vi "7SegmentDecoder.vi"() -> ()   [LabVIEW 2022 SP3]
panel:
  out "DH":T1 {"E" scale=0.0..1.0 scale format="%b"; "D" scale=0.0..1.0 scale format="%b"; "C" scale=0.0..1.0 scale format="%b"; "G" scale=0.0..1.0 scale format="%b"; "B" scale=0.0..1.0 scale format="%b"; "A" scale=0.0..1.0 scale format="%b"; "F" scale=0.0..1.0 scale format="%b"}
  out "UH":T1 {"E" scale=0.0..1.0 scale format="%b"; "D" scale=0.0..1.0 scale format="%b"; "C" scale=0.0..1.0 scale format="%b"; "G" scale=0.0..1.0 scale format="%b"; "B" scale=0.0..1.0 scale format="%b"; "A" scale=0.0..1.0 scale format="%b"; "F" scale=0.0..1.0 scale format="%b"}
  out "DM":T1 {"E" scale=0.0..1.0 scale format="%b"; "D" scale=0.0..1.0 scale format="%b"; "C" scale=0.0..1.0 scale format="%b"; "G" scale=0.0..1.0 scale format="%b"; "B" scale=0.0..1.0 scale format="%b"; "A" scale=0.0..1.0 scale format="%b"; "F" scale=0.0..1.0 scale format="%b"}
  out "UM":T1 {"E" scale=0.0..1.0 scale format="%b"; "D" scale=0.0..1.0 scale format="%b"; "C" scale=0.0..1.0 scale format="%b"; "G" scale=0.0..1.0 scale format="%b"; "B" scale=0.0..1.0 scale format="%b"; "A" scale=0.0..1.0 scale format="%b"; "F" scale=0.0..1.0 scale format="%b"}
  out "DS":T1 {"E" scale=0.0..1.0 scale format="%b"; "D" scale=0.0..1.0 scale format="%b"; "C" scale=0.0..1.0 scale format="%b"; "G" scale=0.0..1.0 scale format="%b"; "B" scale=0.0..1.0 scale format="%b"; "A" scale=0.0..1.0 scale format="%b"; "F" scale=0.0..1.0 scale format="%b"}
  in  "stop":bool
  out "US":T1 {"E" scale=0.0..1.0 scale format="%b"; "D" scale=0.0..1.0 scale format="%b"; "C" scale=0.0..1.0 scale format="%b"; "G" scale=0.0..1.0 scale format="%b"; "B" scale=0.0..1.0 scale format="%b"; "A" scale=0.0..1.0 scale format="%b"; "F" scale=0.0..1.0 scale format="%b"}
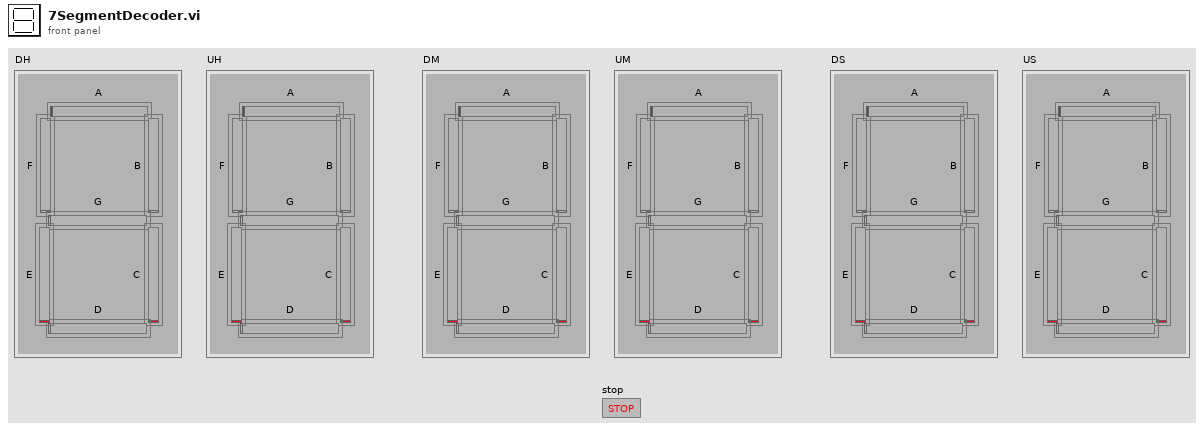
[diagram p1: front panel]
types:
  T1 = cluster{"F":u8, "A":u8, "B":u8, "G":u8, "C":u8, "D":u8, "E":u8}
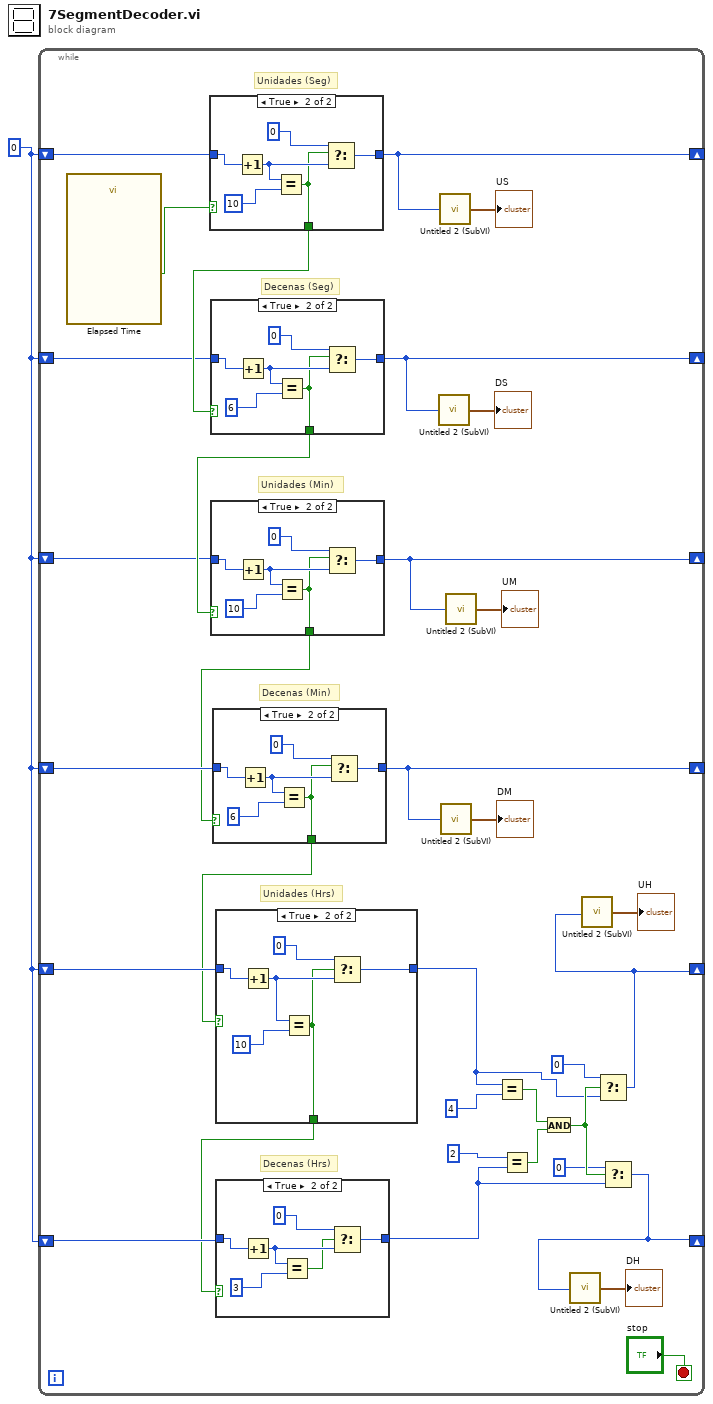
[diagram p0: block diagram]
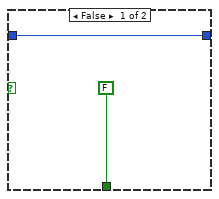
[diagram p3: hidden frame]
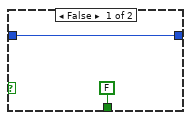
[diagram p4: hidden frame]
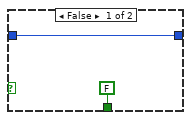
[diagram p5: hidden frame]
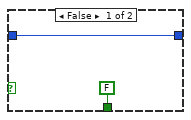
[diagram p6: hidden frame]
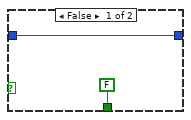
[diagram p7: hidden frame]
diagram:
  w1 = 0
  n1 = while {
    shift-right: [w31] -> _
    shift-left: w1 -> [w32]
    shift-right: [w27] -> _
    shift-left: w1 -> [w29]
    shift-right: [w23] -> _
    shift-left: w1 -> [w25]
    shift-right: [w20] -> _
    shift-left: w1 -> [w21]
    shift-right: [w5] -> _
    shift-left: w1 -> [w17]
    shift-right: [w4] -> _
    shift-left: w1 -> [w14]
    stop <- "stop" stop-if-true
    # "Decenas (Hrs)"
    # "Unidades (Hrs)"
    # "Unidades (Min)"
    # "Decenas (Min)"
    # "Decenas (Seg)"
    # "Unidades (Seg)"
    n2 = call "Elapsed Time"() -> ("Time has Elapsed"=w34:bool)  [unwired: 12 in, 7 out]
    n3 = case shown="True" w34 {
      tunnel: [w76 w79] -> w31
      tunnel: w32 -> [w76 w80]
      tunnel: [FALSE w77] -> w30
      frame False {
      }
      frame True {
        n4 = Increment(x=w80) -> (x+1=w78:i32)
        n5 = Equal?(x=w78, y=10) -> (x = y?=w77:bool)
        n6 = Select(t=0, s=w77, f=w78) -> (s? t:f=w79:i32)
      }
    }
    n7 = case shown="True" w30 {
      tunnel: [w68 w72] -> w27
      tunnel: w29 -> [w68 w70]
      tunnel: [FALSE w69] -> w26
      frame False {
      }
      frame True {
        n8 = Increment(x=w70) -> (x+1=w71:i32)
        n9 = Equal?(x=w71, y=6) -> (x = y?=w69:bool)
        n10 = Select(t=0, s=w69, f=w71) -> (s? t:f=w72:i32)
      }
    }
    n11 = case shown="True" w26 {
      tunnel: [w60 w64] -> w23
      tunnel: w25 -> [w60 w62]
      tunnel: [FALSE w61] -> w19
      frame False {
      }
      frame True {
        n12 = Increment(x=w62) -> (x+1=w63:i32)
        n13 = Equal?(x=w63, y=10) -> (x = y?=w61:bool)
        n14 = Select(t=0, s=w61, f=w63) -> (s? t:f=w64:i32)
      }
    }
    n15 = case shown="True" w19 {
      tunnel: [w52 w56] -> w20
      tunnel: w21 -> [w52 w54]
      tunnel: [FALSE w53] -> w16
      frame False {
      }
      frame True {
        n16 = Increment(x=w54) -> (x+1=w55:i32)
        n17 = Equal?(x=w55, y=6) -> (x = y?=w53:bool)
        n18 = Select(t=0, s=w53, f=w55) -> (s? t:f=w56:i32)
      }
    }
    n19 = case shown="True" w16 {
      tunnel: [w43 w46] -> w3
      tunnel: w17 -> [w43 w48]
      tunnel: [FALSE w45] -> w13
      frame False {
      }
      frame True {
        n20 = Increment(x=w48) -> (x+1=w47:i32)
        n21 = Equal?(x=w47, y=10) -> (x = y?=w45:bool)
        n22 = Select(t=0, s=w45, f=w47) -> (s? t:f=w46:i32)
      }
    }
    n23 = case shown="True" w13 {
      tunnel: [w36 w40] -> w2
      tunnel: w14 -> [w36 w38]
      frame False {
      }
      frame True {
        n24 = Increment(x=w38) -> (x+1=w39:i32)
        n25 = Equal?(x=w39, y=3) -> (x = y?=w37:bool)
        n26 = Select(t=0, s=w37, f=w39) -> (s? t:f=w40:i32)
      }
    }
    n27 = call "Untitled 2 (SubVI).vi"("Numeric"=w27) -> ("Cluster"=→"DS":T1)
    n28 = call "Untitled 2 (SubVI).vi"("Numeric"=w31) -> ("Cluster"=→"US":T1)
    n29 = call "Untitled 2 (SubVI).vi"("Numeric"=w20) -> ("Cluster"=→"DM":T1)
    n30 = call "Untitled 2 (SubVI).vi"("Numeric"=w23) -> ("Cluster"=→"UM":T1)
    n31 = Equal?(x=w3, y=4) -> (x = y?=w9:bool)
    n32 = Equal?(x=2, y=w2) -> (x = y?=w10:bool)
    n33 = And(x=w9, y=w10) -> (x .and. y?=w7:bool)
    n34 = Select(t=0, s=w7, f=w3) -> (s? t:f=w5:i32)
    n35 = call "Untitled 2 (SubVI).vi"("Numeric"=w5) -> ("Cluster"=→"UH":T1)
    n36 = Select(t=0, s=w7, f=w2) -> (s? t:f=w4:i32)
    n37 = call "Untitled 2 (SubVI).vi"("Numeric"=w4) -> ("Cluster"=→"DH":T1)
  }
